vi "Handle getAll.vi"(8 "error in (no error)":errorcluster, 11 "instrument.PPMS3 in":refnum<class "instrument.PPMS3.lvclass">) -> (0 "error out":errorcluster, 2 "getAll":variant, 3 "instrument.PPMS out":refnum<class "instrument.PPMS3.lvclass">)   [LabVIEW 2019, in "instrument.PPMS3.lvclass"]
uses:
  instrument.PPMS3.lvclass
  C:/Users/patrick/Documents/GitHub/PPMS-Monitor-and-Control/lvsrc/instrument.PPMS/instrument.PPMS.lvclass
  instrument.PPMS/Typedefs/PPMS.getAll--cluster.ctl
  instrument.PPMS/instrument.PPMS.lvclass
  C:/Program Files (x86)/National Instruments/LabVIEW 2019/user.lib/LevyLab/Instrument Framework/Instrument Types/Cryostat/Instrument.Cryostat.lvclass
  C:/Program Files (x86)/National Instruments/LabVIEW 2019/user.lib/LevyLab/Instrument Framework/SMOs/Instrument/Instrument.lvclass
  C:/Program Files (x86)/National Instruments/LabVIEW 2019/vi.lib/JKI/JKI SMO/SMO/SMO.lvclass
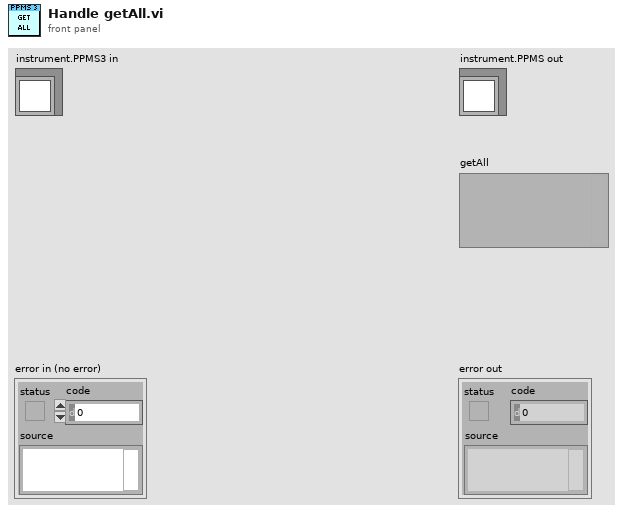
[diagram p1: front panel]
types:
  T1 = typedef "instrument.PPMS.lvclass/PPMS.getAll--cluster.ctl" = cluster{"Chamber Status":string, "Helium Level (%)":dbl, "Temperature (K)":dbl, "Temperature Status":string, "Magnetic Field (T)":dbl, "Magnet Status":string, "Position (°)":dbl}
  T2 = typedef "instrument.PPMS.lvclass/PPMS.Temperature Status--cluster.ctl" = cluster{"Temperature (K)":dbl, "Temperature Status":string}
  T3 = typedef "instrument.PPMS.lvclass/PPMS.Magnet Status--cluster.ctl" = cluster{"Field (T)":dbl, "Magnet Status":string}
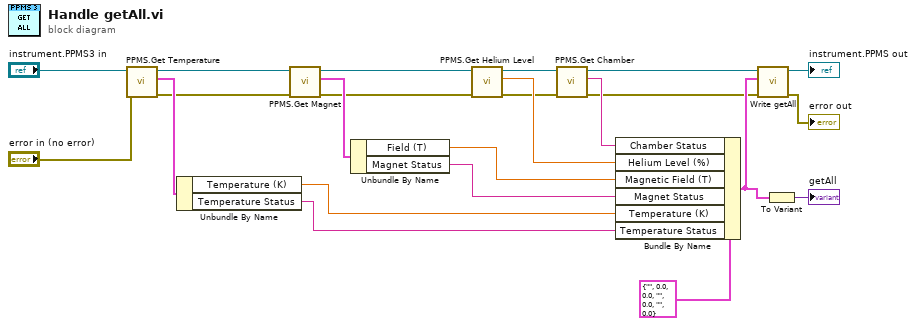
[diagram p0: block diagram]
diagram:
  n1 = call "PPMS.Get Temperature.vi"("error in (no error)"="error in (no error)", "instrument.PPMS"="instrument.PPMS3 in") -> ("error out"=w13:errorcluster, "Temperature Status"=w18:T2, "instrument.PPMS out"=w20:refnum<class "instrument.PPMS3.lvclass">)  [unwired: 7 in]
  n2 = Unbundle By Name(w18) -> ("Temperature (K)"=w17:dbl, "Temperature Status"=w16:string)
  n3 = call "PPMS.Get Magnet.vi"("error in (no error)"=w13, "instrument.PPMS"=w20) -> ("error out"=w12:errorcluster, "Magnet Status"=w15:T3, "instrument.PPMS out"=w19:refnum<class "instrument.PPMS3.lvclass">)  [unwired: 7 in]
  n4 = Unbundle By Name(w15) -> ("Field (T)"=w10:dbl, "Magnet Status"=w11:string)
  n5 = call "PPMS.Get Helium Level.vi"("error in (no error)"=w12, "instrument.PPMS"=w19) -> ("error out"=w7:errorcluster, "Helium Level (%)"=w22:dbl, "instrument.PPMS out"=w8:refnum<class "instrument.PPMS3.lvclass">)  [unwired: 7 in]
  n6 = call "PPMS.Get Chamber.vi"("error in (no error)"=w7, "instrument.PPMS"=w8) -> ("error out"=w3:errorcluster, "Status String"=w6:string, "instrument.PPMS out"=w5:refnum<class "instrument.PPMS3.lvclass">)  [unwired: 7 in]
  n7 = Bundle By Name(cluster=T1 {"Chamber Status"="", "Helium Level (%)"=0.0, "Temperature (K)"=0.0, "Temperature Status"="", "Magnetic Field (T)"=0.0, "Magnet Status"="", "Position (°)"=0.0} ("getAll"), "Chamber Status"=w6, "Helium Level (%)"=w22, "Magnetic Field (T)"=w10, "Magnet Status"=w11, "Temperature (K)"=w17, "Temperature Status"=w16) -> (w4:T1)
  n8 = call "Write getAll.vi"("error in (no error)"=w3, "getAll"=w4, "instrument.PPMS in"=w5) -> ("error out"=→"error out":errorcluster, "instrument.PPMS out"=→"instrument.PPMS out":refnum<class "instrument.PPMS3.lvclass">)  [unwired: 7 in]
  n9 = To Variant(anything=w4) -> (Variant=→"getAll":variant)
